vi "Find Max Font Size.vi"(6 "alignment(left, top)":T3, 8 "String":string, 9 "Text origin(0,0)":cluster{"horizontal":i16, "vertical":i16}, 10 "Bounding Rect":T1, 11 "Font In":T2) -> (1 "Text Bounding Rect":T1, 3 "Font Out":T2)   [LabVIEW 2012, in "String XControl.xctl"]
uses:
  String XControl.xctl
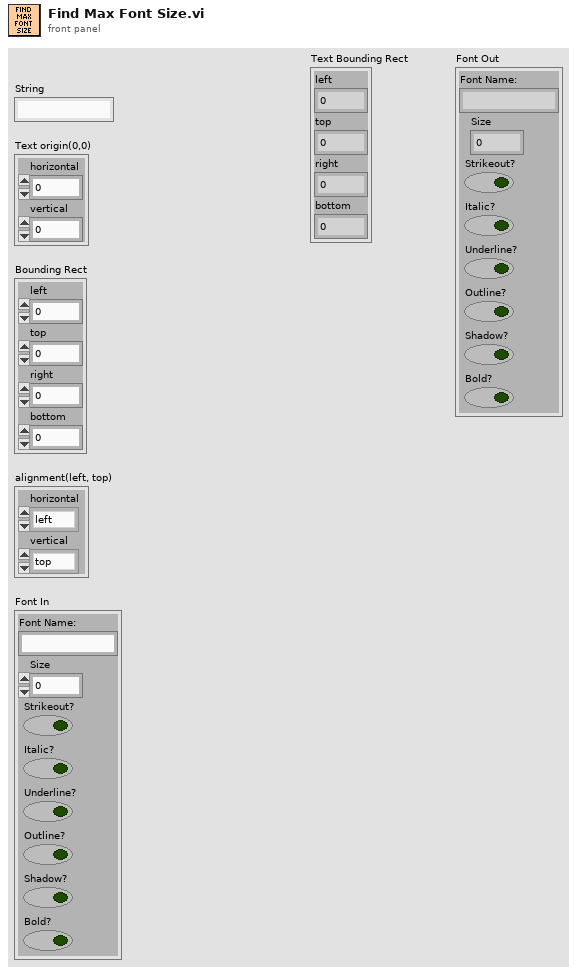
[diagram p1: front panel]
types:
  T1 = cluster{"left":i16, "top":i16, "right":i16, "bottom":i16}
  T2 = cluster{"Font Name:":string, "Size":i16, "Strikeout?":bool, "Italic?":bool, "Underline?":bool, "Outline?":bool, "Shadow?":bool, "Bold?":bool}
  T3 = cluster{"horizontal":enum16{"left", "center", "right"}, "vertical":enum16{"top", "center", "bottom"}}
  T4 = enum16{"User-specified Font", "Application Font", "System Font", "Dialog Font"}
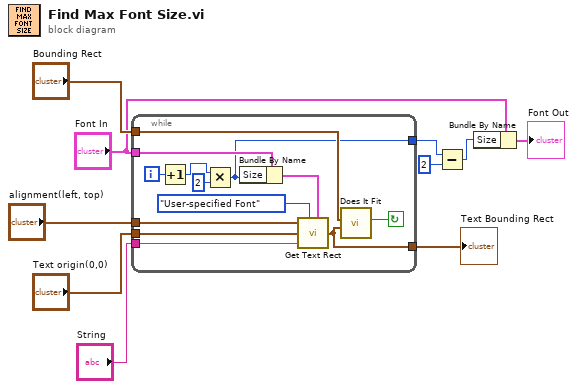
[diagram p0: block diagram]
diagram:
  n1 = while {
    tunnel: "Font In" -> [w18]
    tunnel: "String" -> [w23]
    tunnel: "Text origin(0,0)" -> [w22]
    tunnel: "alignment(left, top)" -> [w21]
    tunnel: "Bounding Rect" -> [w20]
    tunnel: [w11] -> w3
    tunnel: [w15] -> w4
    i -> [w13]
    stop <- w19 continue-if-true
    n2 = Increment(x=w13) -> (x+1=w12:i32)
    n3 = Multiply(x=w12, y=2) -> (x*y=w11:i32)
    n4 = Bundle By Name(cluster=w18, "Size"=w11) -> (w17:T2)
    n5 = call <vilib>:"Get Text Rect.vi"("alignment(left, top)"=w21, "desired font(Application)"=T4."User-specified Font", "origin(0,0)"=w22, "text"=w23, "[user-specified font]"=w17) -> ("rect"=w15:T1)  [unwired: 4 in]
    n6 = call "Does It Fit.vi"("Inner Rect"=w15, "Outer Rect"=w20) -> ("Fit?"=w19:bool)  [unwired: 9 in]
  }
  "Text Bounding Rect" <- w4
  n7 = Subtract(x=w3, y=2) -> (x-y=w2:i32)
  n8 = Bundle By Name(cluster="Font In", "Size"=w2) -> (→"Font Out":T2)
